vi "Odour_map_selection.vi"(10 "NewVal":i32, 11 "Odour component data":T1) -> (2 "Array":dbl[](array[numeric]), 3 "Array 2":dbl[](array[numeric]))   [LabVIEW 2016]
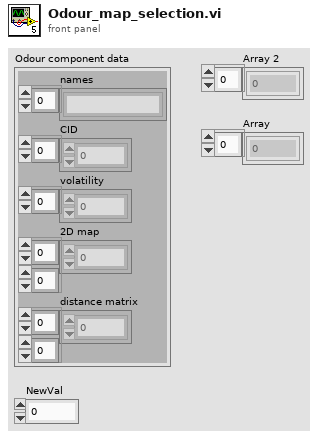
[diagram p1: front panel]
types:
  T1 = cluster{"names":string[], "CID":i32[], "volatility":dbl[], "2D map":dbl[][], "distance matrix":dbl[][]}
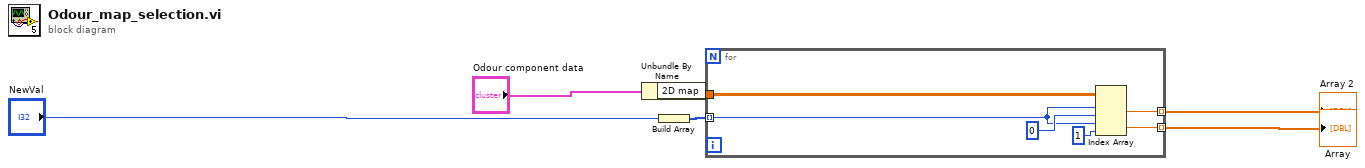
[diagram p0: block diagram]
diagram:
  n1 = Unbundle By Name("Odour component data") -> ("2D map"=w3:dbl[][])
  n2 = Build Array("NewVal") -> (w6:i32[])
  n3 = for {
    tunnel: w3 -> [w12]
    tunnel: [w11] -> w4 mode=indexing
    tunnel: [w10] -> w5 mode=indexing
    tunnel: w6 -> [w8] mode=indexing
    n4 = Index Array(array=w12, index (row) #1=w8, index (col) #1=0 ("disabled index (col)"), index (row) #2=w8, index (col) #2=1 ("disabled index (col)")) -> (element #1=w11:dbl, element #2=w10:dbl)
  }
  "Array" <- w5
  "Array 2" <- w4
